vi "Create directories.vi"(8 "error in (no error)":errorcluster, 10 "Directories to create":string[](array[string]), 11 "File Transfer Behavior in":refnum<class "File Transfer Behavior.lvclass">) -> (0 "error out":errorcluster, 2 "Directories with errors":string[](array[string]), 3 "File Transfer Behavior out":refnum<class "File Transfer Behavior.lvclass">)   [LabVIEW 2015, in "RT Management.lvlib" / "File Transfer Behavior.lvclass"]
doc: "This is a wrapper for the \"Create directory.vi\" to create multiple directories."
uses:
  File Transfer Behavior.lvclass
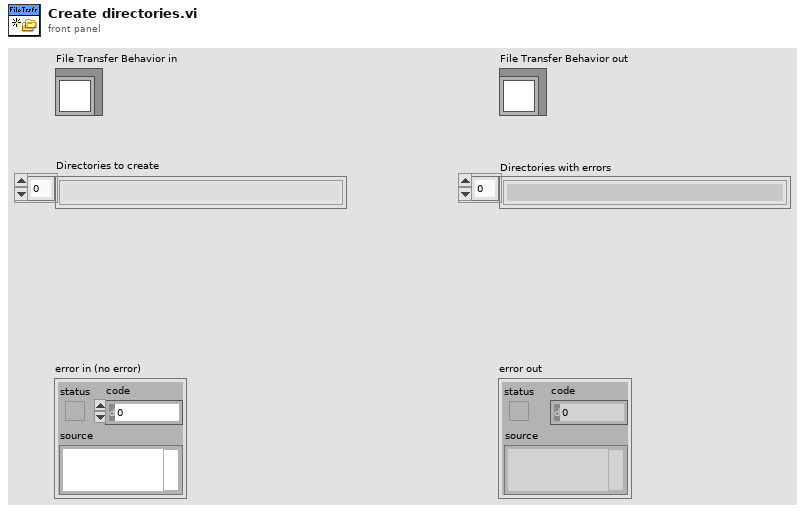
[diagram p1: front panel]
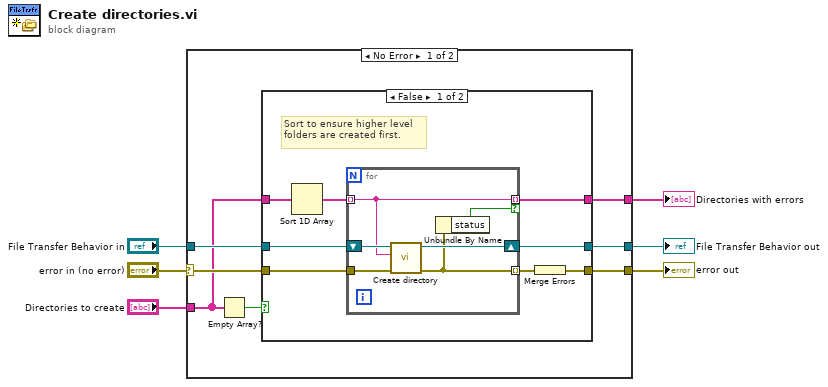
[diagram p0: block diagram]
diagram:
  n1 = case shown="No Error" "error in (no error)" {
    selector: "error in (no error)" -> [w12 w31]
    tunnel: [w11 w31] -> w5
    tunnel: "Directories to create" -> [w7 _]
    tunnel: "File Transfer Behavior in" -> [w9 w30]
    tunnel: [w10 _] -> w1
    tunnel: [w8 w30] -> w4
    frame No Error {
      n2 = Empty Array?(array=w7) -> (empty?=w13:bool)
      n3 = case shown="False" w13 {
        tunnel: [w19 w29] -> w11
        tunnel: w12 -> [w21 w29]
        tunnel: w7 -> [w15 _]
        tunnel: w9 -> [w18 w28]
        tunnel: [w16 _] -> w10
        tunnel: [w17 w28] -> w8
        frame False {
          # "Sort to ensure higher level folders are created first."
          n4 = Sort 1D Array(array=w15) -> (sorted array=w14:string[])
          n5 = for {
            tunnel: [w24] -> w20 mode=indexing
            tunnel: w21 -> [w27]
            tunnel: w14 -> [w23] mode=indexing
            shift-right: [w25] -> w17
            shift-left: w18 -> [w26]
            tunnel: [w23] -> w16 mode=indexing if=w22
            n6 = call-dynamic "Create directory.vi"("error in (no error)"=w27, "Directory"=w23, "File Transfer Behavior in"=w26) -> ("error out"=w24:errorcluster, "File Transfer Behavior out"=w25:refnum<class "File Transfer Behavior.lvclass">)  [unwired: 7 in]
            n7 = Unbundle By Name(w24) -> ("status"=w22:bool)
          }
          n8 = Merge Errors(w20) -> (w19:errorcluster)
        }
        frame True {
        }
      }
    }
    frame Error {
    }
  }
  "error out" <- w5
  "File Transfer Behavior out" <- w4
  "Directories with errors" <- w1
